vi "CRC Check.vi"(10 "subarray":u16[](array[numeric]), 11 "Numeric":i32) -> (3 "Failure Read":u32)   [LabVIEW 2019]
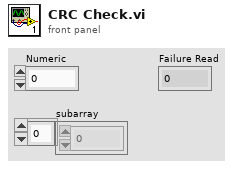
[diagram p1: front panel]
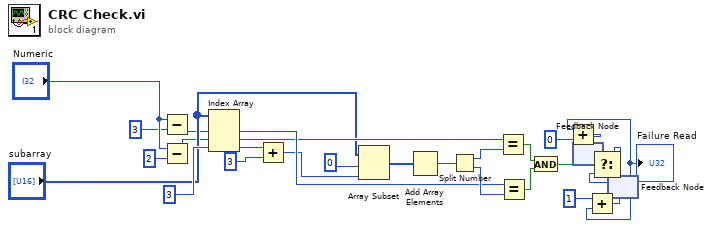
[diagram p0: block diagram]
diagram:
  n1 = Subtract(x="Numeric", y=3) -> (x-y=w1:i32)
  n2 = Subtract(x="Numeric", y=2) -> (x-y=w5:i32)
  n3 = Index Array(array="subarray", index #1=w1, index #2=w5, index #3=3 ("index")) -> (element #1=w16:u16, element #2=w15:u16, element #3=w9:u16)
  n4 = Add(x=w9, y=u16 3) -> (x+y=w11:u16)
  n5 = Array Subset(array="subarray", index=0, length=w11) -> (w12:u16[])
  n6 = Add Array Elements(numeric array=w12) -> (sum=w13:u16)
  n7 = Split Number(x=w13) -> (hi(x)=w14:u8, lo(x)=w17:u8)
  n8 = Equal?(x=w15, y=w14) -> (x = y?=w18:bool)
  n9 = Equal?(x=w16, y=w17) -> (x = y?=w19:bool)
  n10 = And(x=w18, y=w19) -> (x .and. y?=w20:bool)
  n11 = feedback #1() -> (w23:u32)  [unwired: 1 in]
  n12 = feedback #2() -> (w26:u32)  [unwired: 1 in]
  "Failure Read" <- w26
  n13 = Add(x=w26, y=u32 0) -> (x+y=w22:u32)
  n14 = feedback-in #1(w22) -> ()
  n15 = Add(x=u32 1, y=w26) -> (x+y=w24:u32)
  n16 = Select(t=w23, s=w20, f=w24) -> (s? t:f=w25:u32)
  n17 = feedback-in #2(w25) -> ()
